vi "rev 1d arr cont.vi"() -> ()   [LabVIEW 2020]
panel:
  out "o/p j":i32[](array[numeric])
  in  "i":dbl
  out "o/p i":i32[](array[numeric])
  out "Array 5":i32[](array[numeric])
  in  "j":dbl
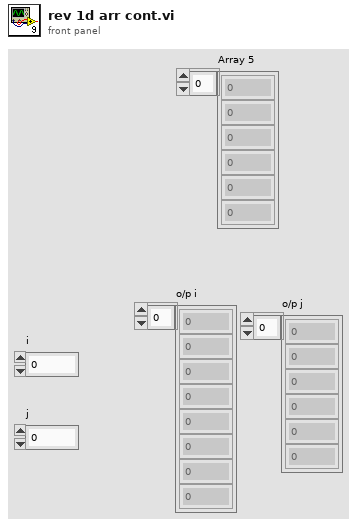
[diagram p1: front panel]
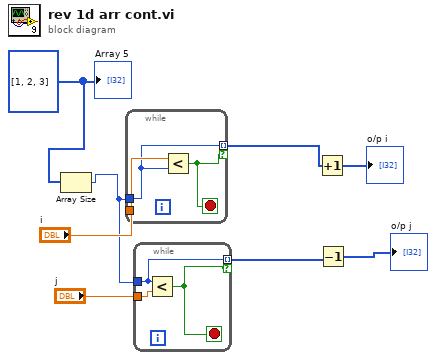
[diagram p0: block diagram]
diagram:
  w6 = i32[] [1, 2, 3]
  n1 = Array Size(array=w6) -> (size(s)=w5:i32)
  n2 = while {
    tunnel: "i" -> [w11]
    tunnel: w5 -> [w10]
    tunnel: [w10] -> w2 mode=indexing if=w9
    stop <- w9 stop-if-true
    n3 = Less?(x=w11, y=w10) -> (x < y?=w9:bool)
  }
  n4 = while {
    tunnel: "j" -> [w14]
    tunnel: w5 -> [w13]
    tunnel: [w13] -> w4 mode=indexing if=w12
    stop <- w12 stop-if-true
    n5 = Less?(x=w13, y=w14) -> (x < y?=w12:bool)
  }
  n6 = Increment(x=w2) -> (x+1=→"o/p i":i32[])
  n7 = Decrement(x=w4) -> (x-1=→"o/p j":i32[])
  "Array 5" <- w6
